vi "CAENHV Get Bd Param Prop Info.vi"(8 "error in (no error)":errorcluster, 9 "ParName":string, 10 "slot":u16, 11 "handle":i32) -> (0 "error out":errorcluster, 2 "PropType":T1, 3 "PropMode":T2)   [LabVIEW 2018, in "CAENHVWrapper.lvlib"]
doc: "CAENHVLIB_API CAENHVRESULT CAENHV_GetBdParamProp(int handle, \n ushort slot, const char *ParName, const char *PropName, void *retval);"
uses:
  <instrlib>/CAENHVWrapper/CAENHVWrapper.lvlib
  <instrlib>/CAENHVWrapper/Types/PARAM_MODE.ctl
  <instrlib>/CAENHVWrapper/Types/PARAM_TYPE.ctl
  <instrlib>/CAENHVWrapper/VIs/CAENHVWrapper.dll
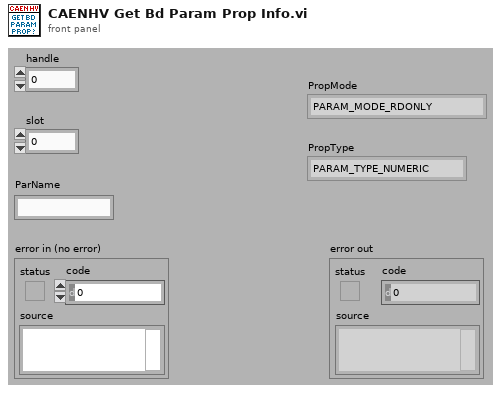
[diagram p1: front panel]
types:
  T1 = typedef "CAENHVWrapper.lvlib/PARAM_TYPE.ctl" = enum32{"PARAM_TYPE_NUMERIC", "PARAM_TYPE_ONOFF", "PARAM_TYPE_CHSTATUS", "PARAM_TYPE_BDSTATUS", "PARAM_TYPE_BINARY", "PARAM_TYPE_STRING"}
  T2 = typedef "CAENHVWrapper.lvlib/PARAM_MODE.ctl" = enum32{"PARAM_MODE_RDONLY", "PARAM_MODE_WRONLY", "PARAM_MODE_RDWR"}
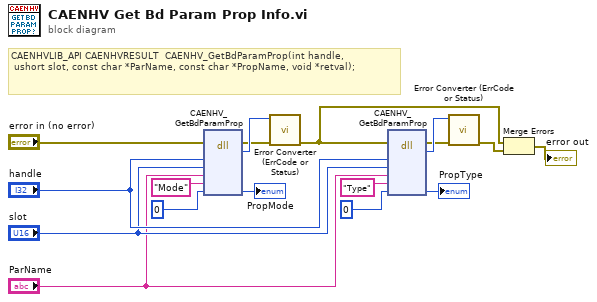
[diagram p0: block diagram]
diagram:
  # "CAENHVLIB_API CAENHVRESULT  CAENHV_GetBdParamProp(int handle, \n ushort slot, const char *ParName, const char *PropName, void *retval);"
  n1 = dll-call lib="C:/Program Files (x86)/National Instruments/LabVIEW 2018/instr.lib/CAENHVWrapper/VIs/CAENHVWrapper.*" fn="CAENHV_GetBdParamProp"(error in="error in (no error)", "handle"="handle", "slot"="slot", "ParName"="ParName", "PropName"="Mode", "retval"=u32 0) -> (error out=w15:errorcluster, "return type"=w16:i32, "retval"=→"PropMode":u32)  [unwired: 6 in, 1 out]
  n2 = call <instrlib>:"Error Converter (ErrCode or Status).vi"("error in (no error)"=w15, "error code"=w16) -> ("error out"=w1:errorcluster)  [unwired: 9 in]
  n3 = dll-call lib="C:/Program Files (x86)/National Instruments/LabVIEW 2018/instr.lib/CAENHVWrapper/VIs/CAENHVWrapper.*" fn="CAENHV_GetBdParamProp"(error in=w1, "handle"="handle", "slot"="slot", "ParName"="ParName", "PropName"="Type", "retval"=u32 0) -> (error out=w7:errorcluster, "return type"=w8:i32, "retval"=→"PropType":u32)  [unwired: 6 in, 1 out]
  n4 = call <instrlib>:"Error Converter (ErrCode or Status).vi"("error in (no error)"=w7, "error code"=w8) -> ("error out"=w6:errorcluster)  [unwired: 9 in]
  n5 = Merge Errors(w1, w6) -> (→"error out":errorcluster)
